vi "Launcher.vi"   [LabVIEW 2020]
uses:
  Libraries/UI/UI.lvlib
types:
  T1 = typedef "UI.lvlib/Broadcast Events--cluster.ctl" = cluster{"Module Did Init":refnum<user-event>, "Status Updated":refnum<user-event>, "Error Reported":refnum<user-event>, "Module Did Stop":refnum<user-event>, "Update Module Execution Status":refnum<user-event>}
  T2 = enum32{"Invalid", "Standard", "Closed", "Hidden", "Minimized", "Maximized"}
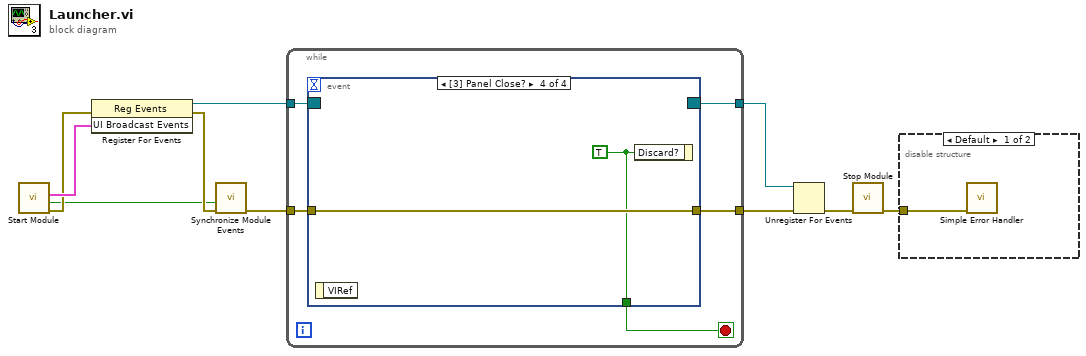
[diagram p0: block diagram]
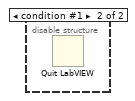
[diagram p2: hidden frame]
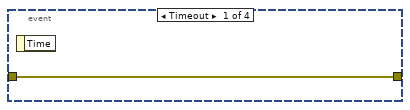
[diagram p3: hidden frame]
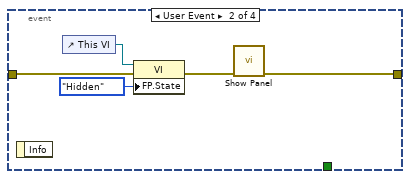
[diagram p4: hidden frame]
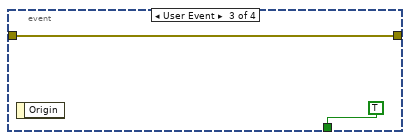
[diagram p5: hidden frame]
diagram:
  n1 = call "Start Module.vi"() -> ("error out"=w9:errorcluster, "Wait for Event Sync?"=w7:bool, "UI Broadcast Events"=w10:T1)  [unwired: 7 in, 2 out]
  n2 = register-events(error in=w9, w10) -> (reference out=w1:refnum<event-registration>, error out=w8:errorcluster)  [unwired: 1 in]
  n3 = call "Synchronize Module Events.vi"("error in"=w8, "Wait for Event Sync?"=w7) -> ("error out"=w6:errorcluster)  [unwired: 9 in]
  n4 = while {
    tunnel: w6 -> [w15]
    tunnel: [w14] -> w5
    tunnel: [w12] -> w2
    tunnel: w1 -> [w11]
    stop <- w13 stop-if-true
    n5 = event shown="[3] Panel Close?" {
      selector: w11 -> [_ _ _ _]
      dyn-events: [_ _ _ _] -> w12
      timeout: _ -> [_ _ _ _]
      tunnel: w15 -> [w16 w19 w23 w25]
      tunnel: [w16 w21 w23 w25] -> w14
      tunnel: [_ _ TRUE ("Discard?") w24] -> w13
      event Timeout {
        n6 = event-data() -> ()  [unwired: 1 in, 1 out]
      }
      event User Event {
        n7 = event-data() -> ()  [unwired: 1 in, 1 out]
        n8 = control-ref of="This VI"() -> (w20:refnum<vi>)
        n9 = property class="VI"(reference=w20, error in=w19, "FP.State"=T2."Hidden" ("Front Panel Window:State")) -> (error out=w18:errorcluster)  [unwired: 1 out]
        n10 = call "Show Panel.vi"("error in"=w18) -> ("error out"=w21:errorcluster)  [unwired: 10 in]
      }
      event User Event {
        n11 = event-data() -> ()  [unwired: 1 in, 1 out]
      }
      event Panel Close? {
        w24 = TRUE ("Discard?")
        n12 = event-data() -> ()  [unwired: 1 in, 1 out]
        n13 = event-data("Discard?"=w24) -> ()  [unwired: 1 in, 1 out]
      }
    }
  }
  n14 = Unregister For Events(event registration refnum=w2, error in=w5) -> (error out=w3:errorcluster)
  n15 = call "Stop Module.vi"("error in"=w3) -> ("error out"=w4:errorcluster)  [unwired: 10 in]
  n16 = disable-structure shown="Default" {
    disable-tunnel: w4 -> [w26 _]
    frame condition #0 (active) {
      n17 = call <vilib>:"Simple Error Handler.vi"("error in (no error)"=w26) -> ()  [unwired: 4 in, 5 out]
    }
    frame condition #1 {
      n18 = Quit LabVIEW() -> ()  [unwired: 1 in]
    }
  }
